vi "Командное слово (SubVI).vi"(6 "Признак команды":bool, 7 "Кол-во слов (1-32)":u8=32, 8 "Команда управления":T1(ring), 9 "Подадрес (1-30)":u8=1, 10 "Разряд прием\\передача":bool, 11 "адрес ОУ (0-30)":u8=1) -> (2 "КС":bool[](array[boolean]))   [LabVIEW 2015]
panel:
  # "4"
  # "7"
  # "5"
  # "6"
  # "8"
  # "11"
  # "20"
  # "9"
  # "10"
  # "12"
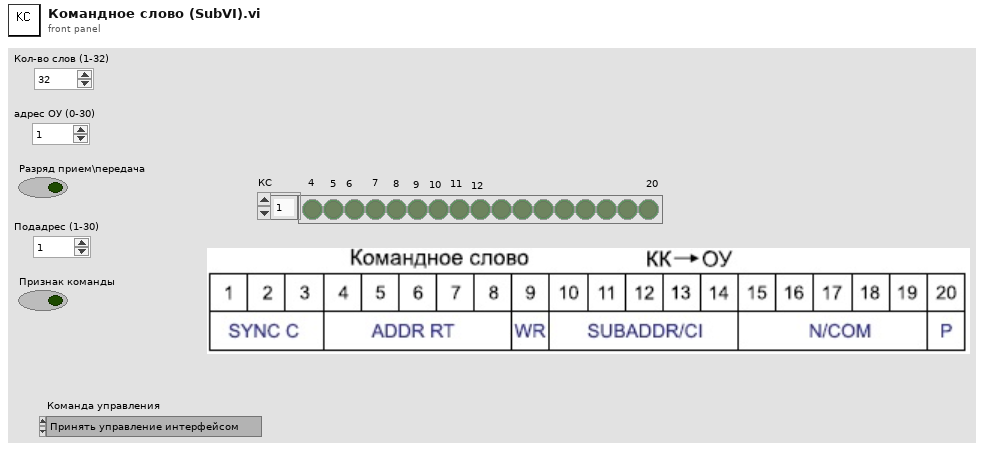
[diagram p1: front panel]
types:
  T1 = enum16{"Принять управление интерфейсом", "Синхронизация", "Передать ОС", "Начать самоконтроль ОУ", "Блокировать передатчик", "Разблокировать передатчик", "Блокировать признак неисправности ОУ", "Разблокировать признак неисправнотси ОУ", "Установить ОУ в исходное состояние", "Резерв", "Передать векорное слово", "Синхронизвция с СД", "Передать последнюю команду", "Передать слово ВСК ОУ", "Блокировать i-й передатчик", "Разблокировать i-й передатчик", "Резерв 2"}
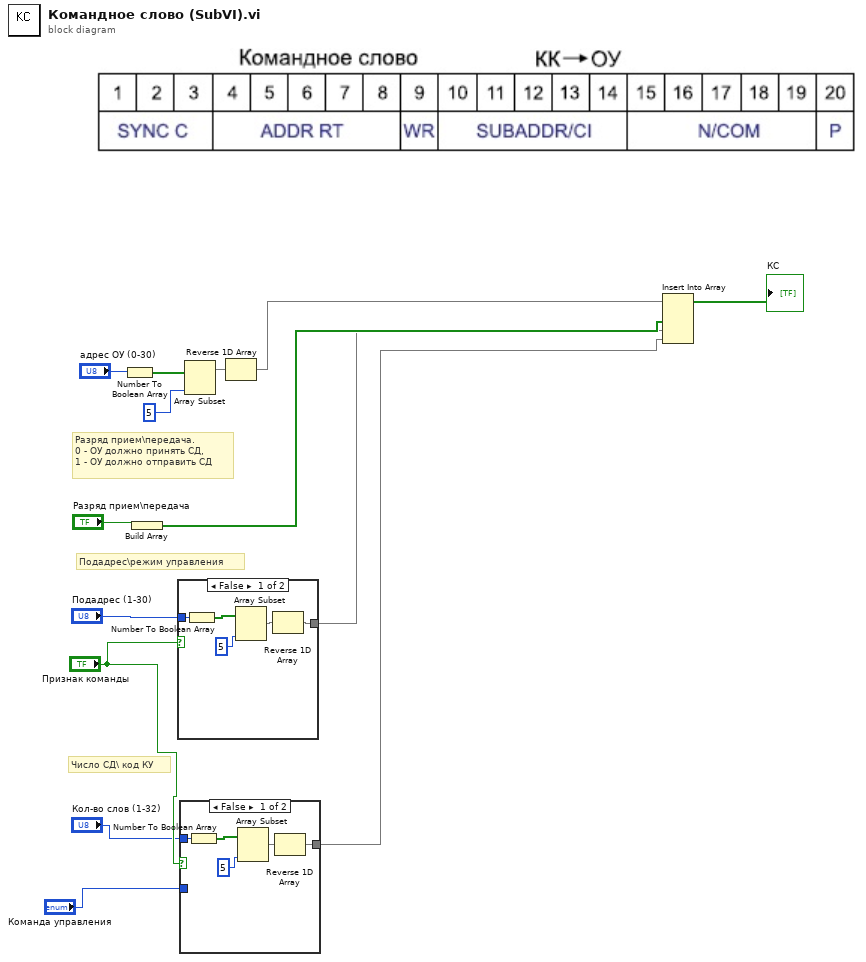
[diagram p0: block diagram]
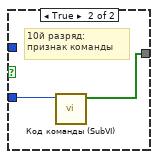
[diagram p2: hidden frame]
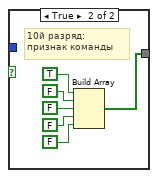
[diagram p3: hidden frame]
diagram:
  # "Подадрес\\режим управления"
  # "Число СД\\ код КУ"
  # "Разряд прием\\передача. \n0 - ОУ должно принять СД,\n1 - ОУ должно отправить СД"
  n1 = Number To Boolean Array(number="адрес ОУ (0-30)") -> (Boolean array=w9:bool[])
  n2 = Build Array("Разряд прием\\передача") -> (w3:bool[])
  n3 = case shown="False" "Признак команды" {
    tunnel: "Подадрес (1-30)" -> [w19 _]
    tunnel: [w15 w20] -> w2
    frame False {
      n4 = Number To Boolean Array(number=w19) -> (Boolean array=w17:bool[])
      n5 = Array Subset(array=w17, length=5) -> (w16:bool[])  [unwired: 1 in]
      n6 = Reverse 1D Array(array=w16) -> (reversed array=w15:bool[])
    }
    frame True {
      # "10й разряд:\nпризнак команды"
      n7 = Build Array(TRUE, FALSE, FALSE, FALSE, FALSE) -> (w20:bool[])
    }
  }
  n8 = case shown="False" "Признак команды" {
    tunnel: "Кол-во слов (1-32)" -> [w30 _]
    tunnel: [w26 w32] -> w1
    tunnel: "Команда управления" -> [_ w31]
    frame False {
      n9 = Number To Boolean Array(number=w30) -> (Boolean array=w28:bool[])
      n10 = Array Subset(array=w28, length=5) -> (w27:bool[])  [unwired: 1 in]
      n11 = Reverse 1D Array(array=w27) -> (reversed array=w26:bool[])
    }
    frame True {
      # "10й разряд:\nпризнак команды"
      n12 = call "Код команды (SubVI).vi"("Команда управления"=w31) -> ("Код команды"=w32:bool[])  [unwired: 10 in]
    }
  }
  n13 = Array Subset(array=w9, length=5) -> (w14:bool[])  [unwired: 1 in]
  n14 = Reverse 1D Array(array=w14) -> (reversed array=w4:bool[])
  n15 = Insert Into Array(array=w4, new element #1=w3, new element #2=w2, new element #3=w1) -> (→"КС":bool[])  [unwired: 1 in]
